vi "Configuration Dialog.vi"(8 "error in (no error)":errorcluster, 11 "Test Runner In":refnum<class "Test Runner.lvclass">) -> (0 "error out":errorcluster, 3 "Test Runner Out":refnum<class "Test Runner.lvclass">)   [LabVIEW 2020, in "Test Runner.lvclass"]
uses:
  Test Runner.lvclass
  C:/Users/anton/Documents/GitHub/LUnit/source/Application Framework/Process Classes/Process/Process.lvclass
  Test Runner.lvclass/Test Runner.ctl
  Application Framework/Support/Configuration File/Configuration File.lvlib
panel:
  in  "Shuffle Test Methods":bool
  in  "Number of Test Runners":u32=2 min=1 step=1
  in  "Cancel":bool
  in  "Commit":bool
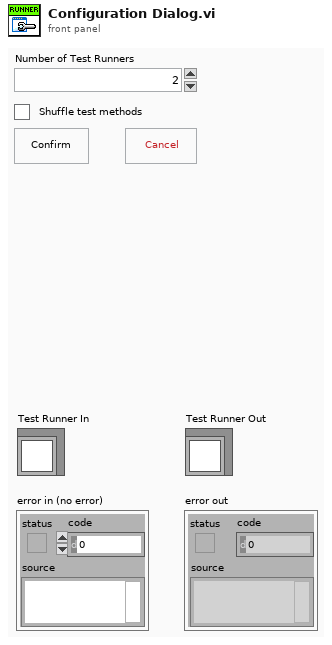
[diagram p1: front panel]
types:
  T1 = typedef "NI_LVConfig.lvlib/Config Data RefNum.ctl" = refnum<k1>
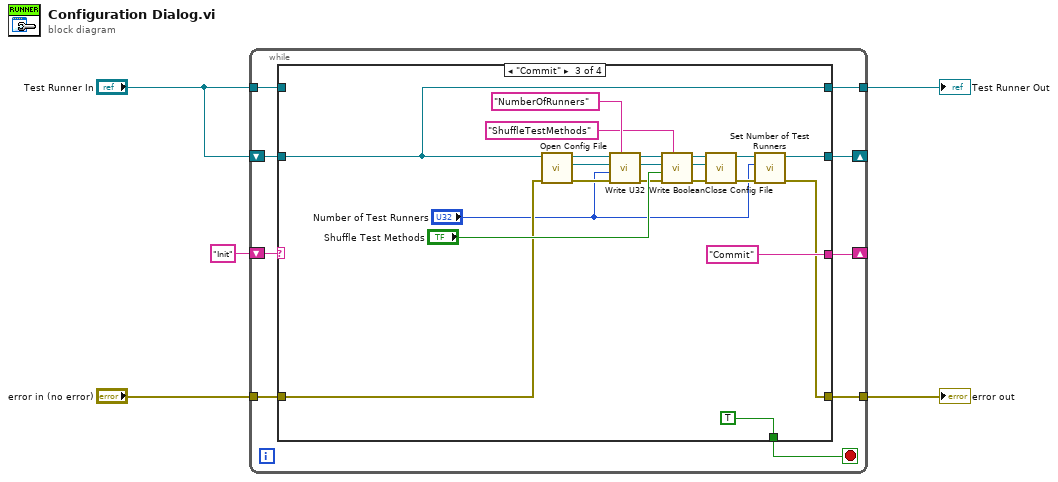
[diagram p0: block diagram]
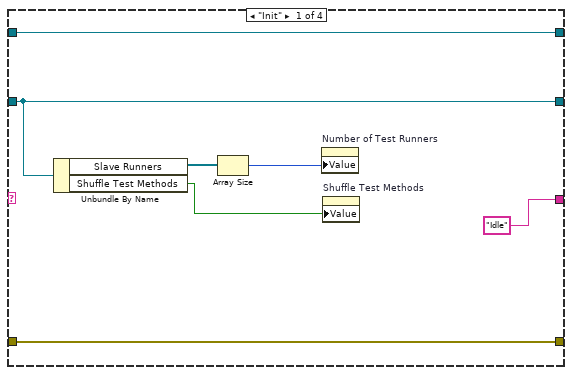
[diagram p2: hidden frame]
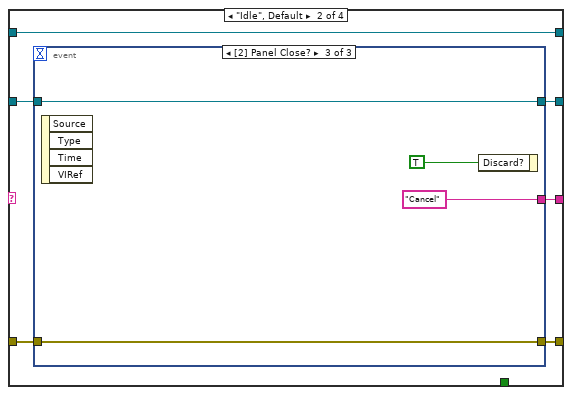
[diagram p3: hidden frame]
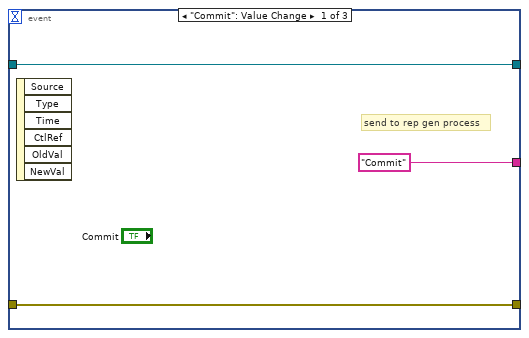
[diagram p4: hidden frame]
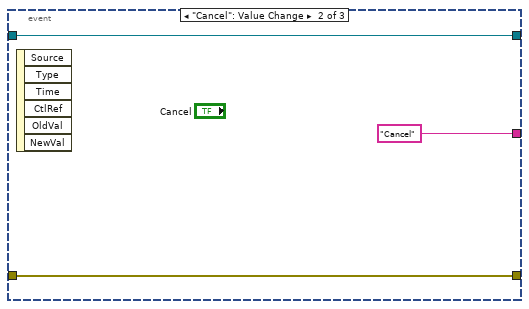
[diagram p5: hidden frame]
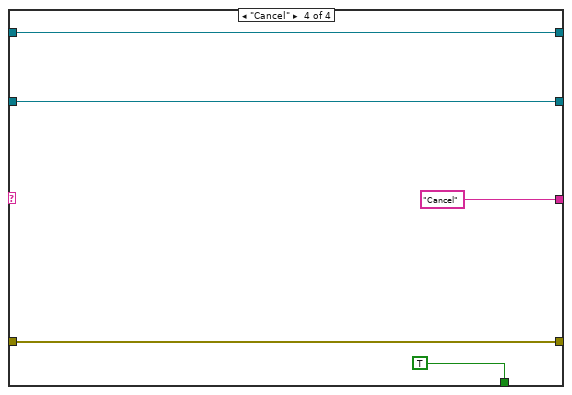
[diagram p6: hidden frame]
diagram:
  n1 = while {
    tunnel: [w14] -> w5
    tunnel: "Test Runner In" -> [w13]
    tunnel: [w12] -> w4
    tunnel: "error in (no error)" -> [w11]
    shift-right: [w8] -> _
    shift-left: "Test Runner In" -> [w9]
    shift-right: [w6] -> _
    shift-left: "Init" -> [w7]
    stop <- w10 stop-if-true
    n2 = case shown="\"Commit\"" w7 {
      tunnel: [w21 w23 w58 w63] -> w14
      tunnel: w13 -> [w21 w23 _ w63]
      tunnel: [w19 w27 w39 w59] -> w12
      tunnel: w11 -> [w19 w26 w48 w59]
      tunnel: [_ _ TRUE TRUE] -> w10
      tunnel: w9 -> [w18 w25 w58 w62]
      tunnel: [w18 w24 w41 w62] -> w8
      tunnel: ["Idle" w22 "Commit" "Cancel"] -> w6
      frame "Init" {
        n3 = Unbundle By Name(w18) -> ("Slave Runners"=w15:refnum<class "Slave Test Runner.lvclass">[], "Shuffle Test Methods"=w16:bool)
        n4 = Array Size(array=w15) -> (size(s)=w17:i32)
        n5 = property on="Number of Test Runners" class="DigNum (strict)"("Value"=w17) -> ()  [unwired: 2 in, 2 out]
        n6 = property on="Shuffle Test Methods" class="Bool (strict)"("Value"=w16) -> ()  [unwired: 2 in, 2 out]
      }
      frame "Idle", Default {
        n7 = event shown="[2] Panel Close?" {
          selector: _ -> [_ _ _]
          dyn-events: _ -> [_ _ _]
          timeout: _ -> [_ _ _]
          tunnel: [w29 w33 w37] -> w27
          tunnel: w26 -> [w29 w33 w37]
          tunnel: w25 -> [w30 w32 w36]
          tunnel: [w30 w32 w36] -> w24
          tunnel: ["Commit" "Cancel" "Cancel"] -> w22
          event "Commit": Value Change {
            # "send to rep gen process"
            n8 = event-data() -> ()  [unwired: 1 in, 6 out]
          }
          event "Cancel": Value Change {
            n9 = event-data() -> ()  [unwired: 1 in, 6 out]
          }
          event Panel Close? {
            n10 = event-data() -> ()  [unwired: 1 in, 4 out]
            n11 = event-data("Discard?"=TRUE) -> ()  [unwired: 1 in, 1 out]
          }
        }
      }
      frame "Commit" {
        n12 = call "Open Config File.vi"("error in (no error)"=w48, "Process in"=w58) -> ("error out"=w46:errorcluster, "refnum out"=w47:T1, "Process out"=w49:refnum<class "Test Runner.lvclass">)  [unwired: 6 in, 1 out]
        n13 = call "Write U32.vi"("key"="NumberOfRunners", "error in (no error)"=w46, "default value"="Number of Test Runners", "refnum"=w47, "Process in"=w49) -> ("error out"=w50:errorcluster, "refnum out"=w45:T1, "Process out"=w55:refnum<class "Test Runner.lvclass">)  [unwired: 3 in, 1 out]
        n14 = call "Write Boolean.vi"("key"="ShuffleTestMethods", "error in (no error)"=w50, "default value"="Shuffle Test Methods", "refnum"=w45, "Process in"=w55) -> ("error out"=w43:errorcluster, "refnum out"=w44:T1, "Process out"=w53:refnum<class "Test Runner.lvclass">)  [unwired: 4 in]
        n15 = call "Close Config File.vi"("error in (no error)"=w43, "refnum"=w44, "Process in"=w53) -> ("error out"=w40:errorcluster, "Process out"=w42:refnum<class "Test Runner.lvclass">)  [unwired: 6 in, 1 out]
        n16 = call "Set Number of Test Runners.vi"("error in (no error)"=w40, "Number of Test Runners"="Number of Test Runners", "Test Runner in"=w42) -> ("error out"=w39:errorcluster, "Test Runner out"=w41:refnum<class "Test Runner.lvclass">)  [unwired: 7 in]
      }
      frame "Cancel" {
      }
    }
  }
  "error out" <- w4
  "Test Runner Out" <- w5
